vi "I2C Write.vi"(5 "EOF":T1, 7 "I2C Channel":u8=1, 8 "Error In":errorcluster, 9 "Data":u8[](array[numeric])=[0], 10 "I2C Slave Address (0)":u8, 11 "LINX Resource":T2={"Platform"=enum."LINX", "Interface"=enum."TCP", "LINX Device Config"={"Interface"=enum."TCP", "COM Port"="N/A", "TCP Configuration"={"IP Address"="panicattack", "Port"=6999}, "Device Family"=4, "Device ID"=1, "Device Name"="Raspberry Pi Model B", "TCP Ref"=refnum, "Channels"={"DI"=[2, 3, 4, 7, 8, 9, 10, 11, 14, 15, 17, 18, 22, 23, 24, 25, 27], "DO"=[2, 3, 4, 7, 8, 9, 10, 11, 14, 15, 17, 18, 22, 23, 24, 25, 27], "AI"=[], "AO"=[], "PWM"=[], "QE"=[], "UART"=[0], "I2C 2"=[0, 1], "SPI"=[0], "CAN"=[], "Servo"=[], "AI Ref (V)"=0.0, "AO Ref (V)"=0.0, "AO Resolution (Bits)"=0}}}) -> (0 "Error Out":errorcluster, 3 "LINX Resource":T2={"Platform"=enum."LINX", "Interface"=enum."TCP", "LINX Device Config"={"Interface"=enum."TCP", "COM Port"="N/A", "TCP Configuration"={"IP Address"="panicattack", "Port"=6999}, "Device Family"=4, "Device ID"=1, "Device Name"="Raspberry Pi Model B", "TCP Ref"=refnum, "Channels"={"DI"=[2, 3, 4, 7, 8, 9, 10, 11, 14, 15, 17, 18, 22, 23, 24, 25, 27], "DO"=[2, 3, 4, 7, 8, 9, 10, 11, 14, 15, 17, 18, 22, 23, 24, 25, 27], "AI"=[], "AO"=[], "PWM"=[], "QE"=[], "UART"=[0], "I2C 2"=[0, 1], "SPI"=[0], "CAN"=[], "Servo"=[], "AI Ref (V)"=0.0, "AO Ref (V)"=0.0, "AO Resolution (Bits)"=0}}})   [LabVIEW 2011, in "LMH-LINX.lvlib"]
doc: "Write data to the specified I2C channel."
uses:
  LMH-LINX.lvlib
  Private/Type Defs/LINX Ref.ctl
  Private/Type Defs/Platform.ctl
  Private/Type Defs/Interface.ctl
  Private/Device/Type Defs/LINX Device Config.ctl
  Private/Device/Type Defs/TCP Config.ctl
  Private/Device/Type Defs/Channels.ctl
  Private/Type Defs/Peripherals/I2C/EOF.ctl
  Private/Type Defs/Peripheral.ctl
  Private/Type Defs/Channel FGV States.ctl
  <vilib>/myRIO/Instrument Drivers/Onboard IO/I2C/typedefs/I2C Transfer Rate.ctl
  <vilib>/myRIO/Instrument Drivers/Onboard IO/I2C/typedefs/I2C Configuration.ctl
  <vilib>/myRIO/Common/Instrument Driver Framework/myRIO v1.0/I2C/typedefs/I2C Channels Enum.ctl
  <vilib>/myRIO/Common/Instrument Driver Framework/Utilities/typedefs/Generic FPGA Reference.ctl
  <vilib>/myRIO/Common/Instrument Driver Framework/Utilities/typedefs/myRIO v1.0 Reference.ctl
  <vilib>/myRIO/Common/Instrument Driver Framework/Utilities/typedefs/Hardware Version Enum.ctl
  <vilib>/myRIO/Common/Instrument Driver Framework/Utilities/typedefs/myRIO Generic Hardware Reference.ctl
  <vilib>/myRIO/Instrument Drivers/Onboard IO/I2C/typedefs/I2C Reference.ctl
  Private/Device/Device.lvlib
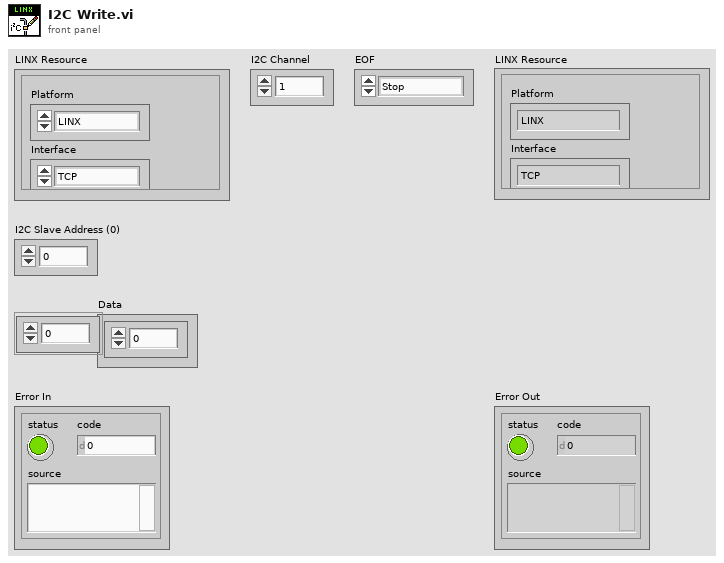
[diagram p1: front panel]
types:
  T1 = typedef "LMH-LINX.lvlib/EOF.ctl" = enum8{"Stop", "Restart", "Restart No Stop", "No Stop"}
  T2 = typedef "LMH-LINX.lvlib/LINX Ref.ctl" = cluster{"Platform":T3, "Interface":T4, "LINX Device Config":T5}
  T3 = typedef "LMH-LINX.lvlib/Platform.ctl" = enum16{"LINX", "myRIO"}
  T4 = typedef "LMH-LINX.lvlib/Interface.ctl" = enum16{"Serial", "TCP"}
  T5 = typedef "LMH-LINX.lvlib/Device.lvlib/LINX Device Config.ctl" = cluster{"Interface":T4, "COM Port":refnum<visa-resource-name>, "TCP Configuration":T6, "Device Family":u8, "Device ID":u8, "Device Name":string, "TCP Ref":refnum<k5>, "Channels":T7}
  T6 = typedef "LMH-LINX.lvlib/Device.lvlib/TCP Config.ctl" = cluster{"IP Address":string, "Port":u16}
  T7 = typedef "LMH-LINX.lvlib/Channels.ctl" = cluster{"DI":u8[], "DO":u8[], "AI":u8[], "AO":u8[], "PWM":u8[], "QE":u8[], "UART":u8[], "I2C 2":u8[], "SPI":u8[], "CAN":u8[], "Servo":u8[], "AI Ref (V)":dbl, "AO Ref (V)":dbl, "AO Resolution (Bits)":u8}
  T8 = typedef "LMH-LINX.lvlib/Peripheral.ctl" = enum8{"DI", "DO", "AI", "AO", "PWM", "QE", "UART", "I2C", "SPI", "CAN", "Servo"}
  T9 = typedef "LMH-LINX.lvlib/Channel FGV States.ctl" = enum16{"Initialize", "Get", "Set"}
  T10 = typedef "I2C.lvlib/I2C Reference.ctl" = cluster{"myRIO Reference":T11, "I2C Channels Enum":T15, "I2C Configuration":T16}
  T11 = typedef "myRIO Generic Hardware Reference.ctl" = cluster{"myRIO Model":T12, "myRIO Hardware Reference":T13}
  T12 = typedef "Hardware Version Enum.ctl" = enum16{"Unknown", "myRIO-1900", "myRIO-1950"}
  T13 = typedef "myRIO v1.0 Reference.ctl" = cluster{"Generic FPGA Reference":T14, "Allow multiple opens":bool}
  T14 = typedef "Generic FPGA Reference.ctl" = refnum<k20>
  T15 = typedef "I2C Channels Enum.ctl" = enum16{"Not Connected", "A/I2C", "B/I2C"}
  T16 = typedef "I2C.lvlib/I2C Configuration.ctl" = cluster{"I2C Transfer Rate":T17}
  T17 = typedef "I2C.lvlib/I2C Transfer Rate.ctl" = enum16{"Standard Mode (100 kbps)", "Fast Mode (400 kbps)"}
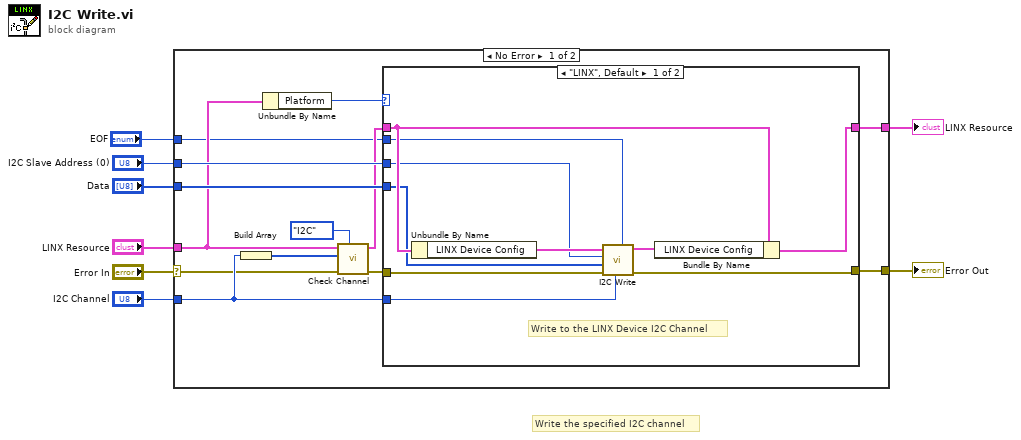
[diagram p0: block diagram]
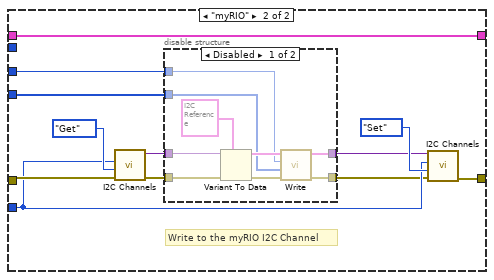
[diagram p2: hidden frame]
diagram:
  # "Write the specified I2C channel"
  n1 = case shown="No Error" "Error In" {
    selector: "Error In" -> [w9 w54]
    tunnel: [w20 w54] -> w8
    tunnel: [w19 w53] -> w7
    tunnel: "Data" -> [w18 _]
    tunnel: "I2C Slave Address (0)" -> [w17 _]
    tunnel: "I2C Channel" -> [w14 _]
    tunnel: "LINX Resource" -> [w12 w53]
    tunnel: "EOF" -> [w10 _]
    frame No Error {
      n2 = Build Array(w14) -> (w13:u8[])
      n3 = Unbundle By Name(w12) -> ("Platform"=w21:T3)
      n4 = call "Check Channel.vi"("Peripheral"=Peripheral."I2C", "Error In"=w9, "Channels"=w13, "LINX Resource"=w12) -> ("Error Out"=w15:errorcluster, "LINX Resource"=w11:T2)  [unwired: 5 in, 1 out]
      n5 = case shown="\"LINX\", Default" w21 {
        tunnel: w15 -> [w28 w39]
        tunnel: w11 -> [w31 w43]
        tunnel: [w29 w42] -> w20
        tunnel: [w30 w43] -> w19
        tunnel: w14 -> [w25 w38]
        tunnel: w18 -> [w23 w34]
        tunnel: w17 -> [w24 w33]
        tunnel: w10 -> [w22 _]
        frame "LINX", Default {
          # "Write to the LINX Device I2C Channel"
          n6 = Unbundle By Name(w31) -> ("LINX Device Config"=w26:T5)
          n7 = call "I2C Write.vi"("EOF"=w22, "I2C Channel (0)"=w25, "Error In"=w28, "Data"=w23, "I2C Slave Address"=w24, "LINX Device Config"=w26) -> ("Error Out"=w29:errorcluster, "LINX Device Config"=w27:T5)  [unwired: 4 in]
          n8 = Bundle By Name(cluster=w31, "LINX Device Config"=w27) -> (w30:T2)
        }
        frame "myRIO" {
          # "Write to the myRIO I2C Channel"
          n9 = call "I2C Channels.vi"("Error In"=w39, "Channel State"=Channel_FGV_States."Get", "Channel Number"=w38) -> ("Error Out"=w37:errorcluster, "I2C Channel"=w35:variant)  [unwired: 7 in]
          n10 = disable-structure shown="Disabled" {
            disable-tunnel: w37 -> [w49 _]
            disable-tunnel: [w48 _] -> w36
            disable-tunnel: w35 -> [w47 _]
            disable-tunnel: w34 -> [w46 _]
            disable-tunnel: w33 -> [w45 _]
            disable-tunnel: [w44 _] -> w32
            frame Disabled {
              n11 = Variant To Data(error in=w49, type=T10 {"myRIO Reference"={"myRIO Model"=enum."Unknown", "myRIO Hardware Reference"={"Generic FPGA Reference"=refnum, "Allow multiple opens"=FALSE}}, "I2C Channels Enum"=enum."Not Connected", "I2C Configuration"={"I2C Transfer Rate"=enum."Standard Mode (100 kbps)"}}, Variant=w47) -> (data=w52:T10, error out=w50:errorcluster)
              n12 = call <vilib>:"Write.vi"("error in (no error)"=w50, "Bytes to Write"=w46, "Slave Address (7-bit)"=w45, "I2C Ref In"=w52) -> ("error out"=w48:errorcluster, "I2C Ref Out"=w44:T10)  [unwired: 6 in]
            }
            frame Enabled {
            }
          }
          n13 = call "I2C Channels.vi"("Error In"=w36, "Channel State"=Channel_FGV_States."Set", "Channel Number"=w38, "I2C Channel"=w32) -> ("Error Out"=w42:errorcluster)  [unwired: 6 in, 1 out]
        }
      }
    }
    frame Error {
    }
  }
  "Error Out" <- w8
  "LINX Resource" <- w7
